vi "Bi_lateralGalvoXYStand_Analog.vi"(8 "error in (no error)":errorcluster, 9 "stand Z vol backforth samp":cluster{"Fs":dbl, "#s":dbl}={"Fs"=500000.0, "#s"=200000.0}, 10 "Bi-Lateral Galvo xy scan range (V)":dbl=0.7 min=0.0 max=1.5, 11 "Bi-Lateral Galvo xy scan frequency (Hz)":i16=500 min=500 max=500) -> (0 "error out":errorcluster, 3 "BiLateralGalvoXYStand":waveform(dbl))   [LabVIEW 2018]
uses:
  <vilib>/measure/NI_MABase.lvlib
panel:
  out "Preview":waveform(dbl)(graph)
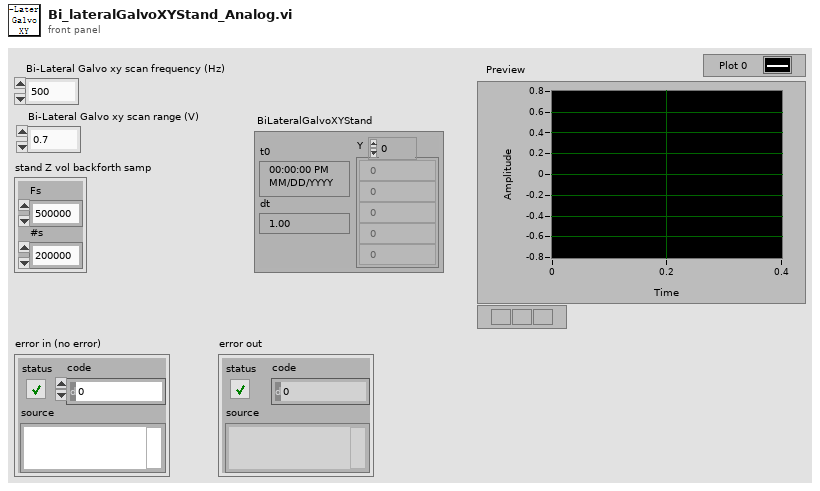
[diagram p1: front panel]
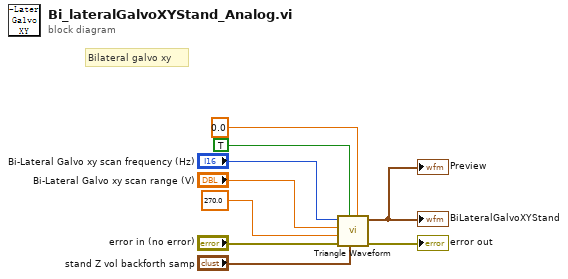
[diagram p0: block diagram]
diagram:
  # "Bilateral galvo xy"
  n1 = call <vilib>:"Triangle Waveform.vi"("offset"=0.0, "sampling info"="stand Z vol backforth samp", "reset signal"=TRUE, "error in (no error)"="error in (no error)", "phase"=270.0, "amplitude"="Bi-Lateral Galvo xy scan range (V)", "frequency"="Bi-Lateral Galvo xy scan frequency (Hz)") -> ("error out"=→"error out":errorcluster, "signal out"=→"BiLateralGalvoXYStand" →"Preview":waveform(dbl))  [unwired: 3 in]
